vi "SetStandbyState.vi"(8 "Error In":errorcluster, 10 "Enable":bool, 11 "Omega CSi32 In":refnum<visa-resource-name>) -> (0 "Error Out":errorcluster, 3 "Omega CSi32 Out":refnum<visa-resource-name>)   [LabVIEW 2012, in "Omega-CSi32.lvlib"]
uses:
  Omega-CSi32.lvlib
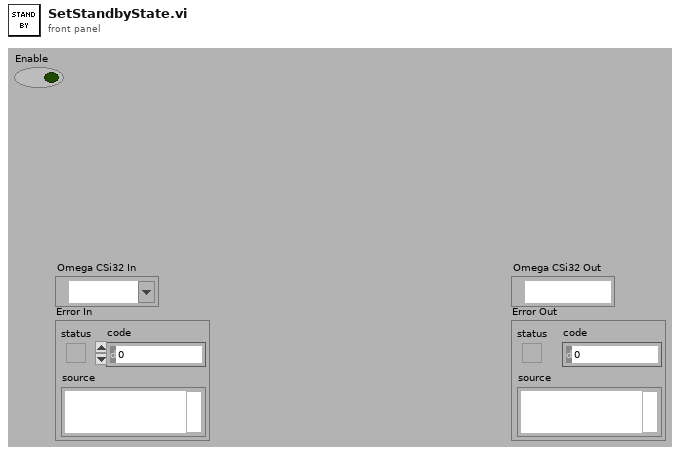
[diagram p1: front panel]
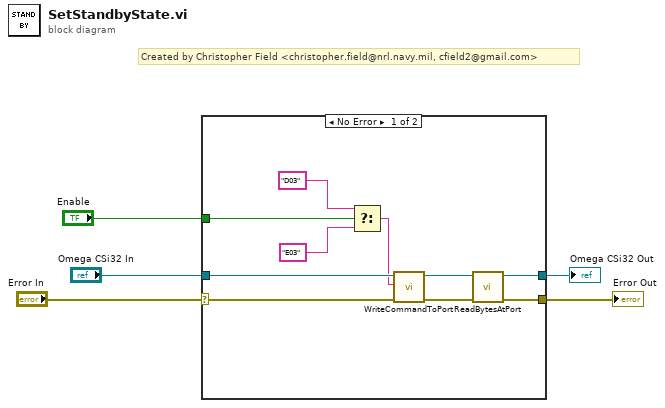
[diagram p0: block diagram]
diagram:
  # "Created by Christopher Field <christopher.field@nrl.navy.mil, cfield2@gmail.com>"
  n1 = case shown="No Error" "Error In" {
    selector: "Error In" -> [w6 w16]
    tunnel: "Omega CSi32 In" -> [w15 w17]
    tunnel: "Enable" -> [w14 _]
    tunnel: [w8 w17] -> w3
    tunnel: [w7 w16] -> w2
    frame No Error {
      n2 = Select(t="D03" ("Command"), s=w14, f="E03" ("Command")) -> (s? t:f=w11:string)
      n3 = call "WriteCommandToPort.vi"("Error In"=w6, "Command"=w11, "CSi32 In"=w15) -> ("Error Out"=w9:errorcluster, "CSi32 Out"=w10:refnum<visa-resource-name>)  [unwired: 7 in]
      n4 = call "ReadBytesAtPort.vi"("Error In"=w9, "CSi32 In"=w10) -> ("Error Out"=w7:errorcluster, "CSi32 Out"=w8:refnum<visa-resource-name>)  [unwired: 7 in, 1 out]
    }
    frame Error {
    }
  }
  "Omega CSi32 Out" <- w3
  "Error Out" <- w2
